vi "Heise Barometric Pressure 901A Send Receive.vi"(8 "error in (no error)":errorcluster, 11 "VISA Refnum in":refnum<visa-resource-name>) -> (0 "error out":errorcluster, 1 "Barometric Data":string[](array[string]), 2 "Barometric Pressure (in Hg)":dbl, 3 "VISA Refnum out":refnum<visa-resource-name>)   [LabVIEW 2016]
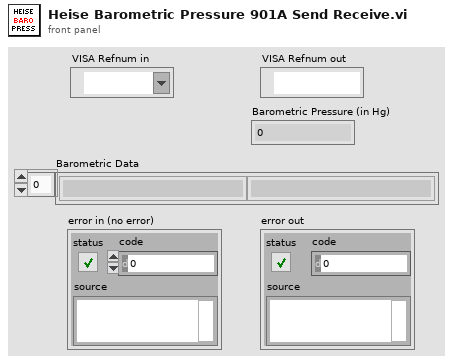
[diagram p1: front panel]
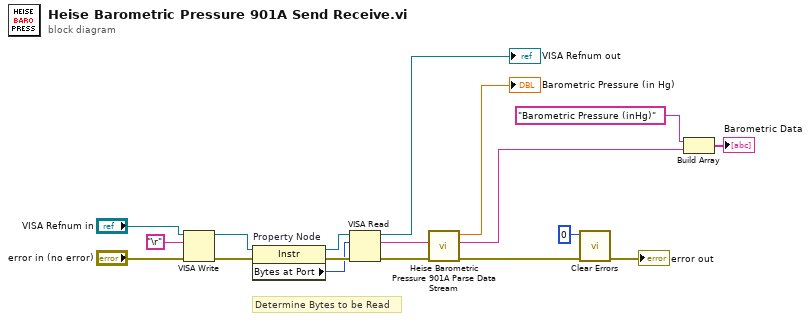
[diagram p0: block diagram]
diagram:
  # "Determine Bytes to be Read"
  n1 = VISA Write(VISA resource name="VISA Refnum in", write buffer="\r", error in (no error)="error in (no error)") -> (VISA resource name out=w16:refnum<visa-resource-name>, error out=w14:errorcluster)  [unwired: 1 out]
  n2 = property on="Property Node" class="Instr"(reference=w16, error in=w14) -> (reference out=w15:refnum<visa-resource-name>, error out=w13:errorcluster, "Bytes at Port"=w12:u32)
  n3 = VISA Read(VISA resource name=w15, byte count=w12, error in (no error)=w13) -> (VISA resource name out=→"VISA Refnum out":refnum<visa-resource-name>, read buffer=w7:string, error out=w8:errorcluster)  [unwired: 1 out]
  n4 = call "Heise Barometric Pressure 901A Parse Data Stream.vi"("Error In"=w8, "Data Stream"=w7) -> ("Error Out"=w2:errorcluster, "Barometric Pressure (in. Hg) String"=w5:string, "Barometric Pressure (in. Hg)"=→"Barometric Pressure (in Hg)":dbl)  [unwired: 7 in]
  n5 = call <vilib>:"Clear Errors.vi"("error in (no error)"=w2, "specific error code to clear (0: all)"=0) -> ("error out"=→"error out":errorcluster)  [unwired: 4 in, 1 out]
  n6 = Build Array("Barometric Pressure (inHg)", w5) -> (→"Barometric Data":string[])
